vi "Patch data preview-Initialise all.vi"() -> (3 "U8 Image ref":T1)   [LabVIEW 2017]
uses:
  <vilib>/vision/Image Controls.llb/IMAQ Image.ctl
  User Interface/Visualisation/Timelapse Viewer/Globals/gl_Time series viewer globals.vi
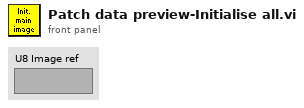
[diagram p1: front panel]
types:
  T1 = typedef "IMAQ Image.ctl" = refnum<image>
  T2 = typedef "Time series viewer refs.ctl" = cluster{"This VI":refnum<vi>, "Image control":refnum<vi>, "AVI Mode ind":refnum<vi>, "Play":refnum<vi>, "Stop":refnum<vi>, "Back":refnum<vi>, "Scrollbar":refnum<vi>, "Video length info":refnum<vi>, "Expected speed values":refnum<vi>, "Intensity":refnum<vi>, "Path":refnum<vi>, "Selection sliders":refnum<vi>, "Speed Graph ref":refnum<vi>, "Frame rate set (fps)":refnum<vi>, "Channel to load":refnum<vi>, "Number of rows to generate":refnum<vi>, "Colour":refnum<vi>}
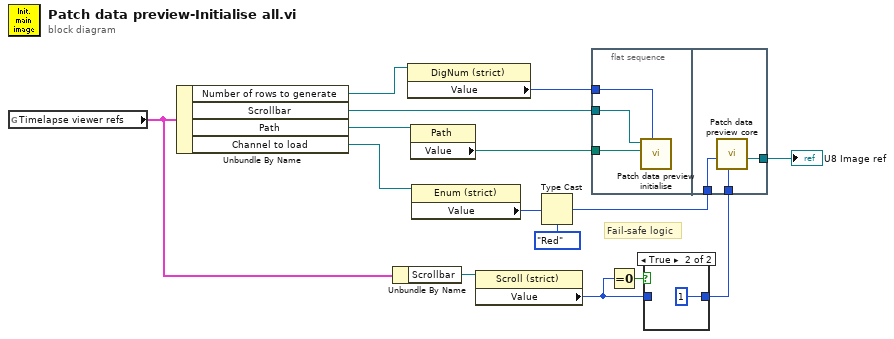
[diagram p0: block diagram]
diagram:
  # "Fail-safe logic"
  n1 = global read "gl_Time series viewer globals.vi" "Timelapse viewer refs"() -> (w4:T2)
  n2 = Unbundle By Name(w4) -> ("Number of rows to generate"=w11:refnum<vi>, "Scrollbar"=w8:refnum<vi>, "Path"=w9:refnum<vi>, "Channel to load"=w13:refnum<vi>)
  n3 = Unbundle By Name(w4) -> ("Scrollbar"=w7:refnum<vi>)
  n4 = property class="DigNum (strict)"(reference=w11) -> ("Value"=w12:i32)  [unwired: 1 in, 2 out]
  n5 = property class="Path"(reference=w9) -> ("Value"=w10:path)  [unwired: 1 in, 2 out]
  n6 = property class="Enum (strict)"(reference=w13) -> ("Value"=w14:enum16{"Show red channel", "Show green channel"})  [unwired: 1 in, 2 out]
  n7 = property class="Scroll (strict)"(reference=w7) -> ("Value"=w2:i32)  [unwired: 1 in, 2 out]
  n8 = Type Cast(type=enum16{"Red", "Green"}."Red" ("Channel to load"), x=w14) -> (*(type *) &x=w6:enum16{"Red", "Green"})
  n9 = flat-sequence {
    tunnel: w12 -> [w18]
    tunnel: w10 -> [w17]
    tunnel: w8 -> [w16]
    tunnel: w6 -> [w21]
    tunnel: w1 -> [w20]
    tunnel: [w19] -> w5
    frame #0 {
      n10 = call "Patch data preview initialise.vi"("Number of rows to generate"=w18, "Dataset path"=w17, "Scrollbar ref"=w16) -> ()  [unwired: 8 in, 1 out]
    }
    frame #1 {
      n11 = call "Patch data preview core.vi"("Global cycle number among all trials"=w20, "Channel to load"=w21) -> ("Image ref (montage)"=w19:T1)  [unwired: 8 in, 1 out]
    }
  }
  n12 = Equal To 0?(x=w2) -> (x = 0?=w3:bool)
  n13 = case shown="True" w3 {
    tunnel: [w22 1 ("Value")] -> w1
    tunnel: w2 -> [w22 _]
    frame False {
    }
    frame True {
    }
  }
  "U8 Image ref" <- w5
